vi "UpdateStateWithRef.vi"(0 "XRef":T9, 1 "Old State":T8, 2 "Version":T6) -> (14 "Is Good?":T5, 15 "Reply":T3, 16 "State Out":T1)   [LabVIEW 2012, in "CRefScripting.lvlib" / "CRef Label Node.xnode"]
doc: "This ability VI is called to perform mutation on an older version of an XNode. If a more recent version of an XNode's library exists, it will be called and let you mutate the old XNode's state appropriately to ensure compatibility with the newer XNode. If you want to report a warning on load of a VI containing an xnode that has its state updated, you can use the reply \"IssueWarning <Custom Load Warning goes here>\". Note that most LV load warnings begin with \"- \", so you will probably want to make yours conform to this standard. The load warning will only be issued if the state is successfully updated.\n\nDefault behavior: None.\n\nThis ability does not provide UI and OS messages are not handled."
uses:
  CRef Label Node.xnode
  <vilib>/XNodeSupport/XNodeXNodeRef.ctl
  <vilib>/XNodeSupport/XNodeVariant.ctl
  <vilib>/XNodeSupport/XNodeVersion.ctl
  <vilib>/XNodeSupport/XNodeUShort.ctl
  <vilib>/XNodeSupport/XNodeBool.ctl
  <vilib>/XNodeSupport/XNodeStringArray.ctl
  <vilib>/XNodeSupport/XNodeString.ctl
  State.ctl
  Core/Master Types.ctl
  <vilib>/XNodeSupport/NI_XNodeSupport.lvlib
  CRef.lvlib
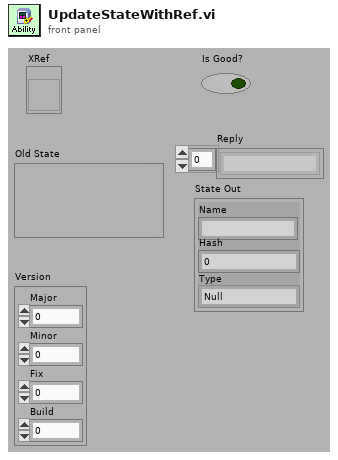
[diagram p1: front panel]
types:
  T1 = typedef "CRefScripting.lvlib/CRef Label Node.xnode/State.ctl" = cluster{"Name":string, "Hash":u32, "Type":T2}
  T2 = typedef "CRef.lvlib/Master Types.ctl" = enum8{"Null", "Boolean", "U8", "I8", "U16", "I16", "U32", "I32", "U64", "I64", "Single", "Double", "Extended", "CSG", "CDB", "CXT", "Boolean(Def)", "U8(Def)", "I8(Def)", "U16(Def)", "I16(Def)", "U32(Def)", "I32(Def)", "Reserved Def", "Reserved Def1", "Single(Def)", "Double(Def)", "Reserved Def2", "Reserved Def3", "Reserved Def4", "Reserved Def5", "Unsigned(Def)", "Signed(Def)", "Real(Def)", "Reserved Def6", "Numeric(Def)", "String"}
  T3 = typedef "NI_XNodeSupport.lvlib/XNodeStringArray.ctl" = T4[]
  T4 = typedef "NI_XNodeSupport.lvlib/XNodeString.ctl" = string
  T5 = typedef "NI_XNodeSupport.lvlib/XNodeBool.ctl" = bool
  T6 = typedef "NI_XNodeSupport.lvlib/XNodeVersion.ctl" = cluster{"Major":T7, "Minor":T7, "Fix":T7, "Build":T7}
  T7 = typedef "NI_XNodeSupport.lvlib/XNodeUShort.ctl" = u16
  T8 = typedef "NI_XNodeSupport.lvlib/XNodeVariant.ctl" = variant
  T9 = typedef "NI_XNodeSupport.lvlib/XNodeXNodeRef.ctl" = refnum<vi>
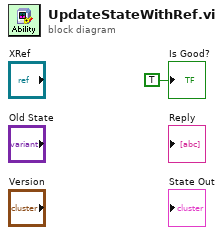
[diagram p0: block diagram]
diagram:
  "Is Good?" <- T5 TRUE ("Is Good?")
